vi "Num To Text_modded.vi"(1 "fmt and prec":T1={"format"=enum."Hex", "precision"=0}, 2 "number":dbl format="%0.2f") -> (0 "numeric string":string)   [LabVIEW 2018]
uses:
  fmt_prec_modded.ctl
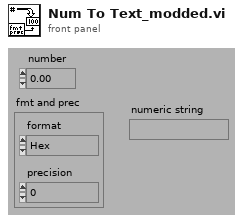
[diagram p1: front panel]
types:
  T1 = typedef "fmt_prec_modded.ctl" = cluster{"format":enum8{"Decimal", "Scientific", "Engineering", "Binary", "Octal", "Hex", "Timestamp"}, "precision":u8}
  T2 = enum8{"Decimal", "Scientific", "Engineering", "Binary", "Octal", "Hex", "Timestamp"}
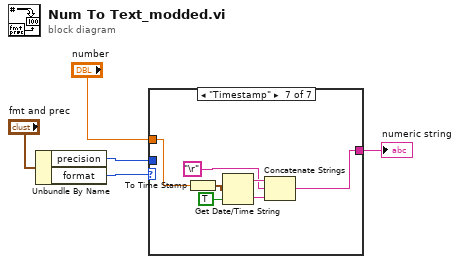
[diagram p0: block diagram]
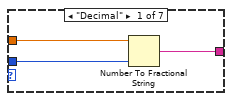
[diagram p2: hidden frame]
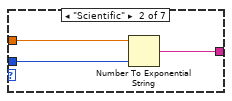
[diagram p3: hidden frame]
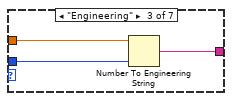
[diagram p4: hidden frame]
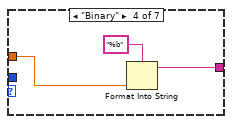
[diagram p5: hidden frame]
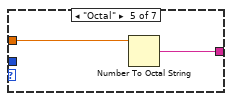
[diagram p6: hidden frame]
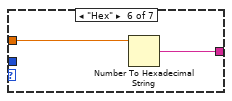
[diagram p7: hidden frame]
diagram:
  n1 = Unbundle By Name("fmt and prec") -> ("precision"=w3:u8, "format"=w1:T2)
  n2 = case shown="\"Timestamp\"" w1 {
    tunnel: [w8 w11 w14 w17 w19 w21 w23] -> w4
    tunnel: w3 -> [w7 w10 w13 _ _ _ _]
    tunnel: "number" -> [w6 w9 w12 w16 w18 w20 w22]
    frame "Decimal" {
      n3 = Number To Fractional String(number=w6, precision (6)=w7) -> (F-format string=w8:string)  [unwired: 2 in]
    }
    frame "Scientific" {
      n4 = Number To Exponential String(number=w9, precision (6)=w10) -> (E-format string=w11:string)  [unwired: 2 in]
    }
    frame "Engineering" {
      n5 = Number To Engineering String(2:w13, 4:w12) -> (0:w14:string)  [unwired: 2 in]
    }
    frame "Binary" {
      n6 = Format Into String(format string="%b", w16) -> (resulting string=w17:string)  [unwired: 2 in, 1 out]
    }
    frame "Octal" {
      n7 = Number To Octal String(2:w18) -> (0:w19:string)  [unwired: 1 in]
    }
    frame "Hex" {
      n8 = Number To Hexadecimal String(2:w20) -> (0:w21:string)  [unwired: 1 in]
    }
    frame "Timestamp" {
      n9 = To Time Stamp(1:w22) -> (0:w28:timestamp)
      n10 = Get Date/Time String(seconds (now)=w28, want seconds? (F)=TRUE) -> (date string=w25:string, time string=w26:string)  [unwired: 1 in]
      n11 = Concatenate Strings(w25, "\r", w26) -> (w23:string)
    }
  }
  "numeric string" <- w4
